vi "myRIO_BRig_FPGA_CueLed.vi"(1 "I_peak":bool, 2 "count":u32, 4 "laser_Npeak":u32=100, 5 "laser_Nvalley":u32=100, 6 "I_CueLed_Event":bool) -> (15 "output_I_peak":bool, 16 "output_count":u32, 18 "output_led":bool)   [LabVIEW 2014]
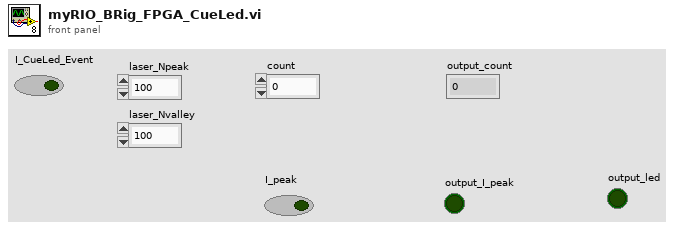
[diagram p1: front panel]
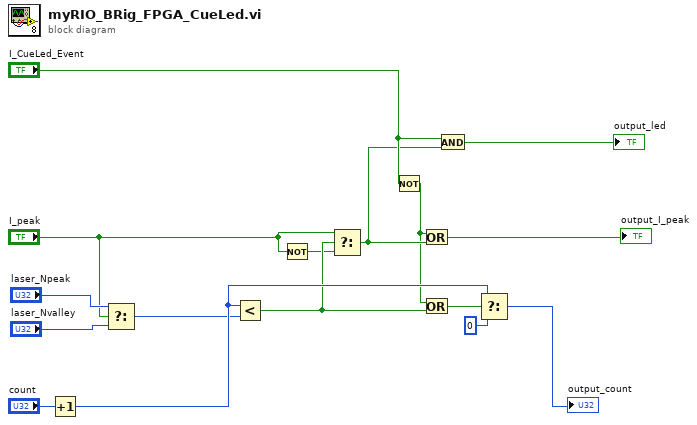
[diagram p0: block diagram]
diagram:
  n1 = Increment(x="count") -> (x+1=w13:u32)
  n2 = Select(t="laser_Npeak", s="I_peak", f="laser_Nvalley") -> (s? t:f=w4:u32)
  n3 = Less?(x=w13, y=w4) -> (x < y?=w3:bool)
  n4 = Not(x="I_peak") -> (.not. x?=w2:bool)
  n5 = Select(t="I_peak", s=w3, f=w2) -> (s? t:f=w6:bool)
  n6 = Not(x="I_CueLed_Event") -> (.not. x?=w5:bool)
  n7 = Or(x=w5, y=w6) -> (x .or. y?=→"output_I_peak":bool)
  n8 = Or(x=w5, y=w3) -> (x .or. y?=w7:bool)
  n9 = And(x="I_CueLed_Event", y=w6) -> (x .and. y?=→"output_led":bool)
  n10 = Select(t=w13, s=w7, f=u32 0) -> (s? t:f=→"output_count":u32)
